vi "Write ITX (2D w X&Y).vi"(4 "Commands":string, 6 "Notes":string, 8 "error in":errorcluster, 9 "Wavenames":cluster{"2D":string, "X":string, "Y":string}, 10 "2D, X, Y (Cluster)":T1, 11 "filename":path) -> (0 "error out":errorcluster, 3 "file out":path)   [LabVIEW 2019, in "LV-Data.ITX.lvclass"]
uses:
  LV-Data.ITX.lvclass
  540a3744-bc28-4862-9360-17f459be1942.vi
  69fdd02c-4d61-444f-9190-9dbe61f219af.vi
  b4ec13a2-1a1e-4ef2-a87f-30a3052f1557.vi
panel:
  out "String":string
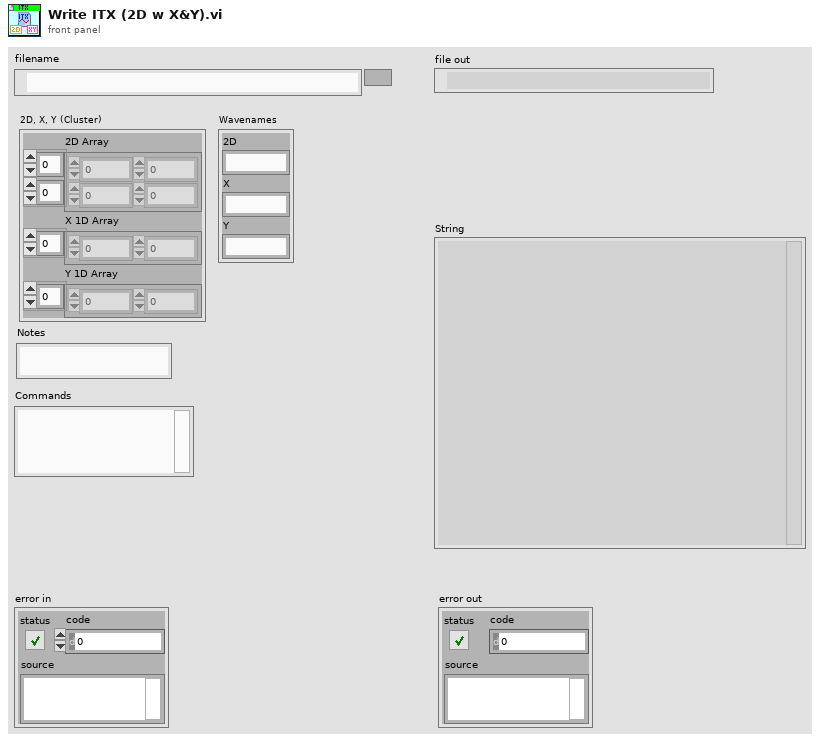
[diagram p1: front panel]
types:
  T1 = cluster{"2D Array":dbl[][], "X 1D Array":dbl[], "Y 1D Array":dbl[]}
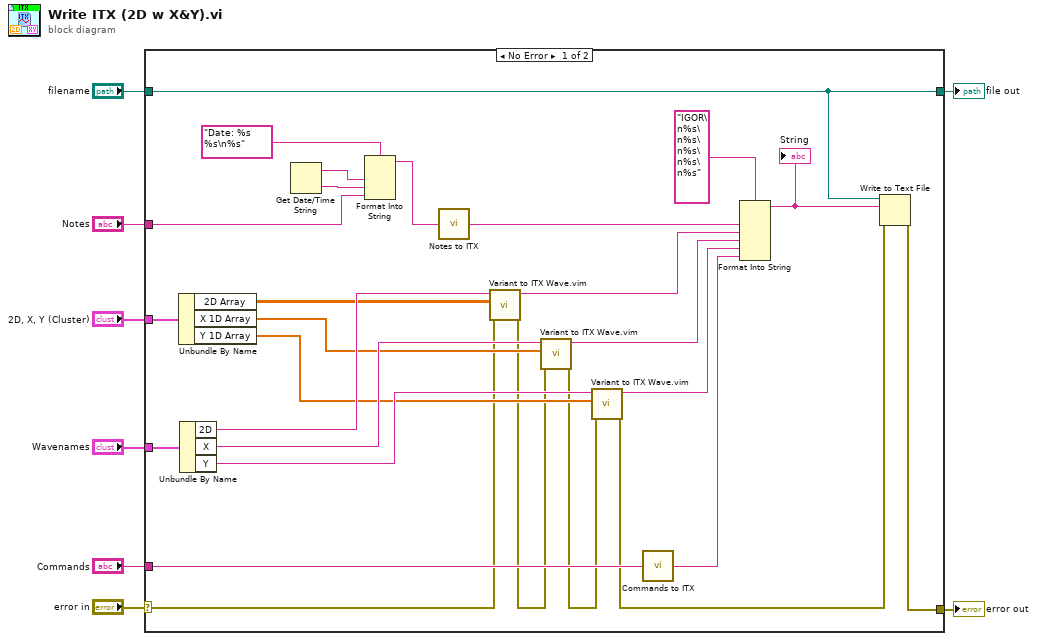
[diagram p0: block diagram]
diagram:
  n1 = case shown="No Error" "error in" {
    selector: "error in" -> [w12 w37]
    tunnel: "Notes" -> [w27 _]
    tunnel: "filename" -> [w34 w36]
    tunnel: "Commands" -> [w22 _]
    tunnel: [w35 w37] -> w4
    tunnel: [w34 w36] -> w3
    tunnel: "2D, X, Y (Cluster)" -> [w33 _]
    tunnel: "Wavenames" -> [w32 _]
    frame No Error {
      n2 = Unbundle By Name(w33) -> ("2D Array"=w20:dbl[][], "X 1D Array"=w17:dbl[], "Y 1D Array"=w14:dbl[])
      n3 = Unbundle By Name(w32) -> ("2D"=w21:string, "X"=w18:string, "Y"=w15:string)
      n4 = Get Date/Time String() -> (date string=w30:string, time string=w31:string)  [unwired: 3 out]
      n5 = Format Into String(format string="Date: %s %s\n%s", w30, w31, w27) -> (resulting string=w28:string)  [unwired: 2 in, 1 out]
      n6 = call "Notes to ITX.vi"("Notes"=w28) -> ("ITX Notes"=w25:string)
      n7 = call "Variant to ITX Wave.vim"("error in (no error)"=w12, "Data"=w20, "Wavename"=w21) -> ("error out"=w9:errorcluster, "ITX Wave"=w19:string)  [unwired: 7 in]
      n8 = call "Variant to ITX Wave.vim"("error in (no error)"=w9, "Data"=w17, "Wavename"=w18) -> ("error out"=w10:errorcluster, "ITX Wave"=w16:string)  [unwired: 7 in]
      n9 = call "Variant to ITX Wave.vim"("error in (no error)"=w10, "Data"=w14, "Wavename"=w15) -> ("error out"=w11:errorcluster, "ITX Wave"=w13:string)  [unwired: 7 in]
      n10 = call "Commands to ITX.vi"("Commands"=w22) -> ("ITX Commands"=w23:string)
      n11 = Format Into String(format string="IGOR\n%s\n%s\n%s\n%s\n%s", w25, w19, w16, w13, w23) -> (resulting string=w24:string)  [unwired: 2 in, 1 out]
      "String" <- w24
      n12 = Write to Text File(file (use dialog)=w34, text=w24, error in=w11) -> (error out=w35:errorcluster)  [unwired: 3 out]
    }
    frame Error {
    }
  }
  "file out" <- w3
  "error out" <- w4
